vi "CmdExe.Generate Measurement based on Exe Return Code.vi"(5 "StdOut is Fail Code":bool, 6 "BaseCode":i32=7000, 7 "Name":string, 8 "Error":errorcluster, 9 "RtnCode":i32, 10 "StdErr":string, 11 "StdOut":string) -> (0 "Success":bool, 3 "Meas":T1 {"Status" items=["LOG", "PASS", "FAIL", "ERROR"]})   [LabVIEW 2018]
uses:
  Results/Result.Measurement Item.ctl
  Results/Result.Measurement and Attribute Item Status.ctl
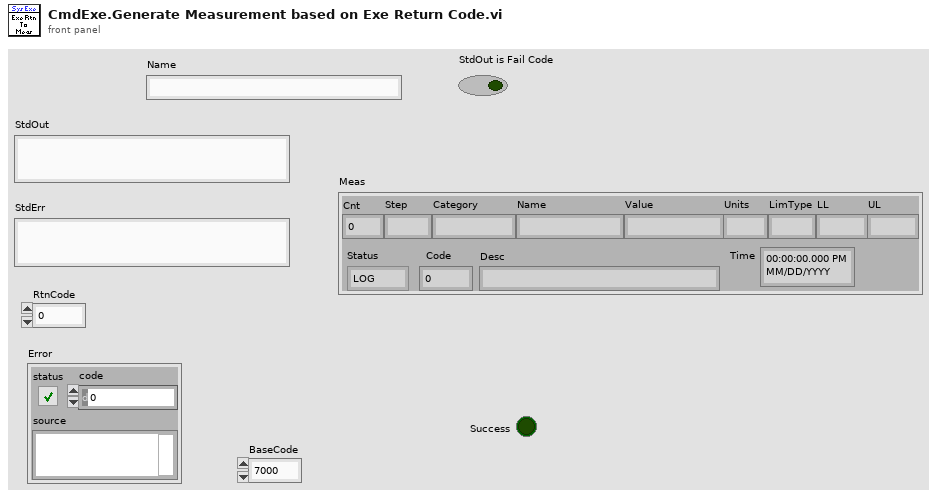
[diagram p1: front panel]
types:
  T1 = typedef "Result.Measurement Item.ctl" = cluster{"Cnt":i32, "Step":string, "Category":string, "Name":string, "Value":string, "Units":string, "LimType":string, "LL":string, "UL":string, "Status":T2, "Code":i32, "Desc":string, "Time":timestamp}
  T2 = typedef "Result.Measurement and Attribute Item Status.ctl" = i32
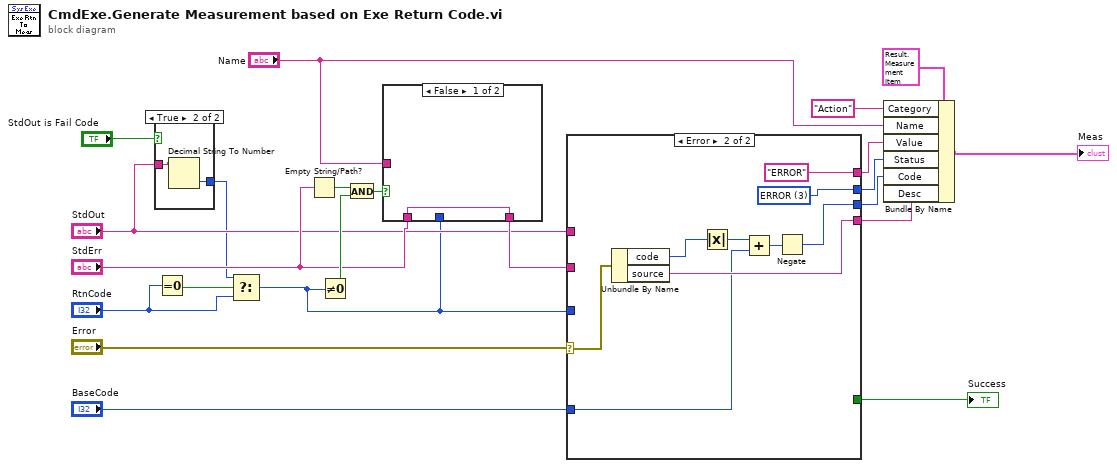
[diagram p0: block diagram]
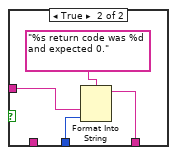
[diagram p3: hidden frame]
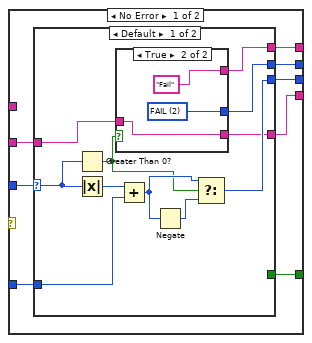
[diagram p4: hidden frame]
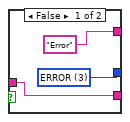
[diagram p5: hidden frame]
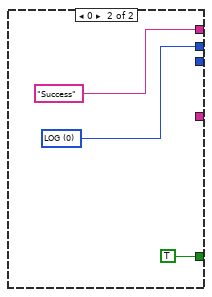
[diagram p6: hidden frame]
diagram:
  n1 = case shown="True" "StdOut is Fail Code" {
    tunnel: "StdOut" -> [_ w24]
    tunnel: [_ w23] -> w4
    frame False {
    }
    frame True {
      n2 = Decimal String To Number(string=w24) -> (number=w23:i32)  [unwired: 2 in, 1 out]
    }
  }
  n3 = Equal To 0?(x="RtnCode") -> (x = 0?=w3:bool)
  n4 = Select(t=w4, s=w3, f="RtnCode") -> (s? t:f=w1:i32)
  n5 = Empty String/Path?(string/path="StdErr") -> (empty?=w12:bool)
  n6 = Not Equal To 0?(x=w1) -> (x != 0?=w11:bool)
  n7 = And(x=w12, y=w11) -> (x .and. y?=w9:bool)
  n8 = case shown="False" w9 {
    tunnel: "StdErr" -> [w25 _]
    tunnel: [w25 w28] -> w8
    tunnel: w1 -> [_ w27]
    tunnel: "Name" -> [_ w26]
    frame False {
    }
    frame True {
      n9 = Format Into String(format string="%s return code was %d and expected 0.", w26, w27) -> (resulting string=w28:string)  [unwired: 2 in, 1 out]
    }
  }
  n10 = case shown="Error" "Error" {
    selector: "Error" -> [_ w65]
    tunnel: [w36 "ERROR"] -> w20
    tunnel: [w37 w63] -> w17
    tunnel: [w32 w58] -> w19
    tunnel: [w30 w64] -> w18
    tunnel: "BaseCode" -> [w33 w60]
    tunnel: "StdOut" -> [_ _]
    tunnel: w8 -> [w34 _]
    tunnel: w1 -> [w35 _]
    tunnel: [w31 _] -> w13
    frame No Error {
      n11 = case shown="Default" w35 {
        selector: w35 -> [w46 _]
        tunnel: [w39 w57] -> w37
        tunnel: [w40 "Success"] -> w36
        tunnel: w34 -> [w41 _]
        tunnel: w33 -> [w47 _]
        tunnel: [w43 _] -> w32
        tunnel: [_ TRUE] -> w31
        tunnel: [w38 _] -> w30
        frame Default {
          n12 = Greater Than 0?(x=w46) -> (x > 0?=w42:bool)
          n13 = Absolute Value(x=w46) -> (abs(x)=w48:i32)
          n14 = case shown="True" w42 {
            tunnel: w41 -> [w49 w52]
            tunnel: ["Error" "Fail"] -> w40
            tunnel: [w50 w53] -> w39
            tunnel: [w49 w52] -> w38
            frame False {
              w50 = T2 3 items=["LOG", "PASS", "FAIL", "ERROR"] ("Status")
            }
            frame True {
              w53 = T2 2 items=["LOG", "PASS", "FAIL", "ERROR"] ("Status")
            }
          }
          n15 = Add(x=w48, y=w47) -> (x+y=w44:i32)
          n16 = Negate(x=w44) -> (-x=w45:i32)
          n17 = Select(t=w44, s=w42, f=w45) -> (s? t:f=w43:i32)
        }
        frame 0 {
          w57 = T2 0 items=["LOG", "PASS", "FAIL", "ERROR"] ("Status")
        }
      }
    }
    frame Error {
      w63 = T2 3 items=["LOG", "PASS", "FAIL", "ERROR"] ("Status")
      n18 = Unbundle By Name(w65) -> ("code"=w62:i32, "source"=w64:string)
      n19 = Absolute Value(x=w62) -> (abs(x)=w61:i32)
      n20 = Add(x=w61, y=w60) -> (x+y=w59:i32)
      n21 = Negate(x=w59) -> (-x=w58:i32)
    }
  }
  "Success" <- w13
  n22 = Bundle By Name(cluster=T1 {"Cnt"=0, "Step"="", "Category"="", "Name"="", "Value"="", "Units"="", "LimType"="", "LL"="", "UL"="", "Status"=0, "Code"=0, "Desc"="", "Time"=timestamp(0 s since 1904-01-01)} ("Meas"), "Category"="Action", "Name"="Name", "Value"=w20, "Status"=w17, "Code"=w19, "Desc"=w18) -> (→"Meas":T1)
